vi "Get Sub Objects Dictionary.vi"(8 "error in":errorcluster, 11 "Object Entry in":refnum<class "Object Entry.lvclass">) -> (0 "error out":errorcluster, 2 "Sub Objects":refnum<class "Sub Objects Dictionary.lvclass">, 3 "Object Entry out":refnum<class "Object Entry.lvclass">)   [LabVIEW 2020, in "CANopen.lvlib" / "Object Entry.lvclass"]
uses:
  Object Entry.lvclass
  Object Entry.lvclass/Object Entry.ctl
  Sub Objects Dictionary/Sub Objects Dictionary.lvclass
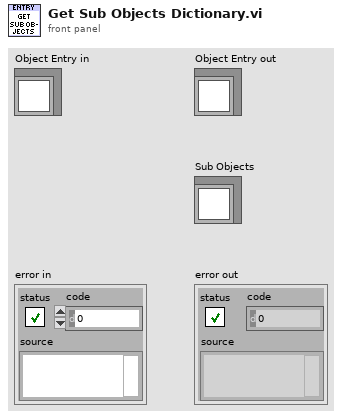
[diagram p1: front panel]
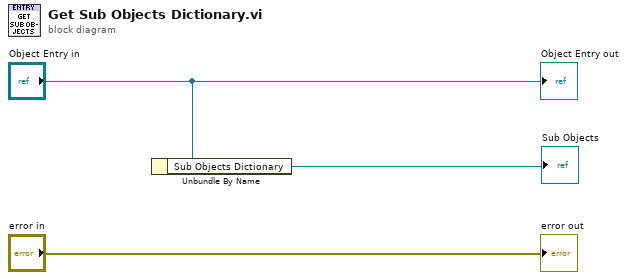
[diagram p0: block diagram]
diagram:
  n1 = Unbundle By Name("Object Entry in") -> ("Sub Objects Dictionary"=→"Sub Objects":refnum<class "Sub Objects Dictionary.lvclass">)
  "error out" <- "error in"
  "Object Entry out" <- "Object Entry in"
